vi "get used disk space.vi"(8 "error in (no error)":errorcluster, 11 "Channel in":refnum<class "Channel.lvclass">) -> (0 "error out":errorcluster, 3 "Channel out":refnum<class "Channel.lvclass">)   [LabVIEW 2018, in "Channel.lvclass"]
uses:
  Channel.lvclass
  Channel.lvclass/Channel.ctl
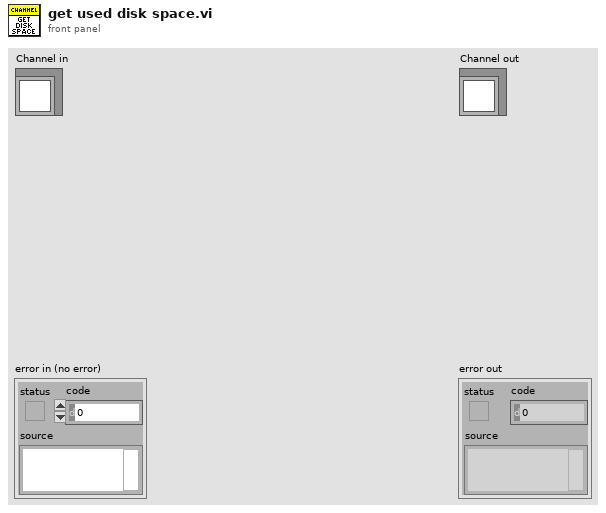
[diagram p1: front panel]
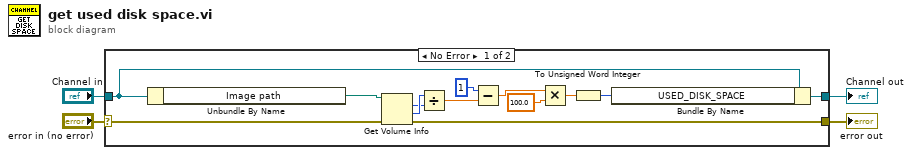
[diagram p0: block diagram]
diagram:
  n1 = case shown="No Error" "error in (no error)" {
    selector: "error in (no error)" -> [w9 w19]
    tunnel: [w8 w19] -> w3
    tunnel: [w6 w18] -> w1
    tunnel: "Channel in" -> [w7 w18]
    frame No Error {
      n2 = Unbundle By Name(w7) -> ("Image path"=w10:path)
      n3 = Get Volume Info(8:w9, 11:w10) -> (0:w8:errorcluster, 1:w17:i64, 2:w16:i64)  [unwired: 3 out]
      n4 = Divide(x=w17, y=w16) -> (x/y=w15:dbl)
      n5 = Subtract(x=1, y=w15) -> (x-y=w13:dbl)
      n6 = Multiply(x=w13, y=100.0) -> (x*y=w11:dbl)
      n7 = To Unsigned Word Integer(number=w11) -> (unsigned 16bit integer=w5:u16)
      n8 = Bundle By Name(cluster=w7, "USED_DISK_SPACE"=w5) -> (w6:refnum<class "Channel.lvclass">)
    }
    frame Error {
    }
  }
  "error out" <- w3
  "Channel out" <- w1
